vi "HexToWord.vi"(11 "数组":u16[](array[numeric]) format="%04xH") -> (3 "WORD":u16[](array[numeric]))   [LabVIEW 2022 SP3, in "挥发酚.lvlib"]
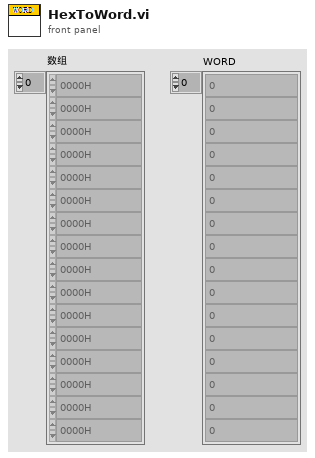
[diagram p1: front panel]
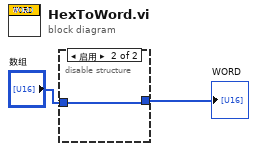
[diagram p0: block diagram]
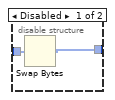
[diagram p2: hidden frame]
diagram:
  n1 = disable-structure shown="启用" {
    disable-tunnel: "数组" -> [w4 w5]
    disable-tunnel: [w3 w5] -> w1
    frame Disabled {
      n2 = Swap Bytes(anything=w4) -> (byte swapped=w3:u16[])
    }
    frame Enabled {
    }
  }
  "WORD" <- w1
